vi "Autonomous Lift Gripper Pickup.vi"(8 "error in (no error)":errorcluster, 11 "Lift References":T19) -> (0 "error out":errorcluster, 3 "Lift References Out":T19)   [LabVIEW 2014]
uses:
  <vilib>/Rock Robotics/WPI/MotorControl/WPI_MotorControlDeviceRef.ctl
  <vilib>/Rock Robotics/WPI/MotorControl/WPI_MotorControlType.ctl
  <vilib>/Rock Robotics/SystemInterfaces/Typedef/FPGA_TypedefDigitalModule.ctl
  <vilib>/Rock Robotics/SystemInterfaces/DIO/FPGA_DIOPWMChannel.ctl
  <vilib>/Rock Robotics/WPI/PWM/WPI_PWMDeadband.ctl
  <vilib>/Rock Robotics/WPI/CAN/Jaguar/SubVIs/WPI_CANJaguar_ControlMode.ctl
  <vilib>/Rock Robotics/WPI/CAN/TalonSRX/WPI_CANTalonSRX_APIControlMode.ctl
  <vilib>/Rock Robotics/WPI/PWM/WPI_PWMTransform_ConPane.ctl
  <vilib>/Rock Robotics/WPI/Potentiometer/WPI_PotentiometerDevRef.ctl
  <vilib>/Rock Robotics/SystemInterfaces/Typedef/FPGA_TypedefAnalogModule.ctl
  <vilib>/Rock Robotics/SystemInterfaces/AI/FPGA_AIChannel.ctl
  <vilib>/Rock Robotics/WPI/Switch/WPI_SwitchDevRef.ctl
  <vilib>/Rock Robotics/SystemInterfaces/DIO/FPGA_DIOChannel.ctl
  <vilib>/Rock Robotics/SystemInterfaces/Counter/FPGA_CounterCtrSystemIndex.ctl
  <vilib>/Rock Robotics/WPI/Encoder/WPI_EncoderDevRef.ctl
  <vilib>/Rock Robotics/SystemInterfaces/Encoder/FPGA_EncoderIdx.ctl
  <vilib>/Rock Robotics/WPI/Encoder/WPI_EncoderType.ctl
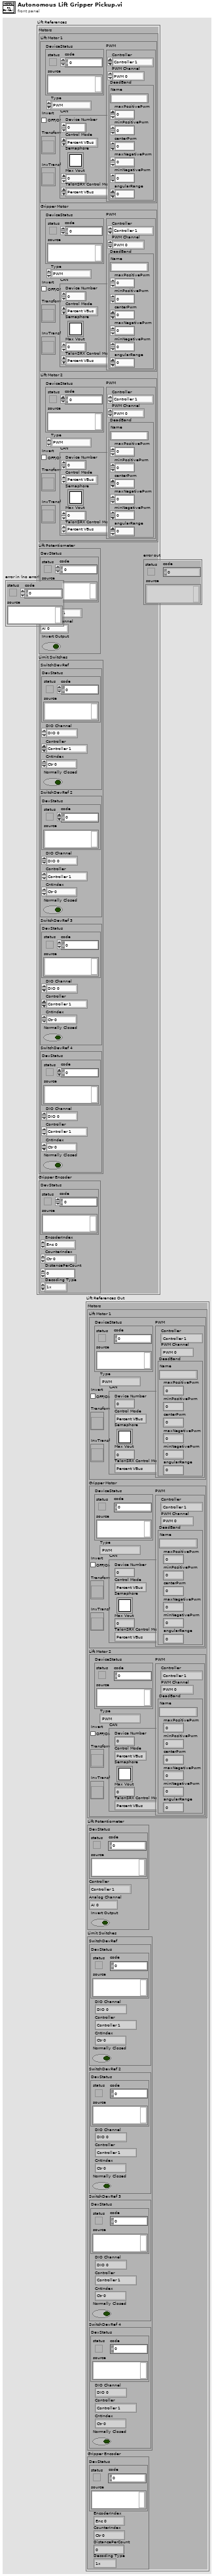
[diagram p1: front panel]
types:
  T1 = typedef "WPI_MotorControlDeviceRef.ctl" = cluster{"DeviceStatus":errorcluster, "Type":T2, "PWM":cluster{"Controller":T3, "PWM Channel":T4, "DeadBand":T5}, "CAN":cluster{"Device Number":u8, "Control Mode":T6, "Semaphore":T7, "Max Vout":dbl, "TalonSRX Control Mode":T8}, "Invert":bool, "TransformRef":T9, "InvTransformRef":T9}
  T2 = typedef "WPI_MotorControlType.ctl" = enum16{"PWM", "CAN", "CANTalonSRX"}
  T3 = typedef "FPGA_TypedefDigitalModule.ctl" = enum16{"Controller 1"}
  T4 = typedef "FPGA_DIOPWMChannel.ctl" = enum8{"PWM 0", "PWM 1", "PWM 2", "PWM 3", "PWM 4", "PWM 5", "PWM 6", "PWM 7", "PWM 8", "PWM 9", "PWM MXP 0", "PWM MXP 1", "PWM MXP 2", "PWM MXP 3", "PWM MXP 4", "PWM MXP 5", "PWM MXP 6", "PWM MXP 7", "PWM MXP 8", "PWM MXP 9", "Invalid"}
  T5 = typedef "WPI_PWMDeadband.ctl" = cluster{"Name":string, "maxPositivePwm":i32, "minPositivePwm":i32, "centerPwm":i32, "maxNegativePwm":i32, "minNegativePwm":i32, "angularRange":u16}
  T6 = typedef "WPI_CANJaguar_ControlMode.ctl" = enum8{"Percent VBus", "Current", "Speed", "Position", "Voltage"}
  T7 = typedef "Semaphore RefNum" = refnum<k1>
  T8 = typedef "WPI_CANTalonSRX_APIControlMode.ctl" = enum8{"Percent VBus", "Speed", "Position", "Slave", "Unchanged / Invalid"}
  T9 = typedef "WPI_PWMTransform_ConPane.ctl" = refnum<vi>
  T10 = typedef "WPI_PotentiometerDevRef.ctl" = cluster{"DevStatus":errorcluster, "Controller":T11, "Analog Channel":T12, "Invert Output":bool}
  T11 = typedef "FPGA_TypedefAnalogModule.ctl" = enum16{"Controller 1"}
  T12 = typedef "FPGA_AIChannel.ctl" = enum8{"AI 0", "AI 1", "AI 2", "AI 3", "AI MXP 0", "AI MXP 1", "AI MXP 2", "AI MXP 3", "Invalid"}
  T13 = typedef "WPI_SwitchDevRef.ctl" = cluster{"DevStatus":errorcluster, "DIO Channel":T14, "Controller":T3, "CntIndex":T15, "Normally Closed":bool}
  T14 = typedef "FPGA_DIOChannel.ctl" = enum8{"DIO 0", "DIO 1", "DIO 2", "DIO 3", "DIO 4", "DIO 5", "DIO 6", "DIO 7", "DIO 8", "DIO 9", "DIO MXP 0", "DIO MXP 1", "DIO MXP 2", "DIO MXP 3", "DIO MXP 4", "DIO MXP 5", "DIO MXP 6", "DIO MXP 7", "DIO MXP 8", "DIO MXP 9", "DIO MXP 10", "DIO MXP 11", "DIO MXP 12", "DIO MXP 13", "DIO MXP 14", "DIO MXP 15", "Invalid"}
  T15 = typedef "FPGA_CounterCtrSystemIndex.ctl" = enum8{"Ctr 0", "Ctr 1", "Ctr 2", "Ctr 3", "Ctr 4", "Ctr 5", "Ctr 6", "Ctr 7", "Invalid"}
  T16 = typedef "WPI_EncoderDevRef.ctl" = cluster{"DevStatus":errorcluster, "EncoderIndex":T17, "CounterIndex":T15, "DistancePerCount":dbl, "Decoding Type":T18}
  T17 = typedef "FPGA_EncoderIdx.ctl" = enum8{"Enc 0", "Enc 1", "Enc 2", "Enc 3", "Enc 4", "Enc 5", "Enc 6", "Enc 7", "Invalid"}
  T18 = typedef "WPI_EncoderType.ctl" = enum16{"1x", "2x", "4x"}
  T19 = cluster{"Motors":cluster{"Lift Motor 1":T1, "Gripper Motor":T1, "Lift Motor 2":T1}, "Lift Potentiometer":T10, "Limit Switches":cluster{"SwitchDevRef":T13, "SwitchDevRef 2":T13, "SwitchDevRef 3":T13, "SwitchDevRef 4":T13}, "Gripper Encoder":T16}
  T20 = cluster{"State Out":enum16{"Normal", "Down/Out", "Down/In", "Up", "Override"}, "To Shift":cluster{"Cluster in":cluster{"Scaled Value Out":dbl, "Distance":dbl}, "To Shift":cluster{"Error":dbl, "millisecond timer value":u32, "To Shift Register":dbl}, "To Shift":dbl}}
  T21 = cluster{"Lift Motor 1":T1, "Gripper Motor":T1, "Lift Motor 2":T1}
  T22 = cluster{"SwitchDevRef":T13, "SwitchDevRef 2":T13, "SwitchDevRef 3":T13, "SwitchDevRef 4":T13}
  T23 = enum16{"Normal", "Down/Out", "Down/In", "Up", "Override"}
  T24 = cluster{"Cluster in":cluster{"Scaled Value Out":dbl, "Distance":dbl}, "To Shift":cluster{"Error":dbl, "millisecond timer value":u32, "To Shift Register":dbl}, "To Shift":dbl}
  T25 = cluster{"Grabber Motor":T1, "Lift Motor 1":T1, "Lift Motor 2":T1}
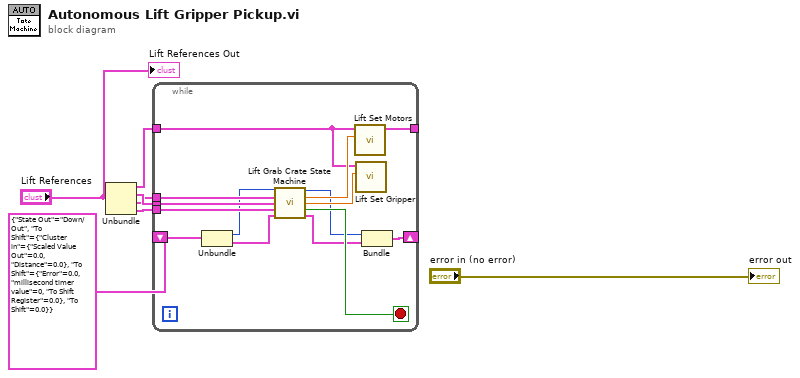
[diagram p0: block diagram]
diagram:
  n1 = Unbundle("Lift References") -> ("Motors"=w7:T21, "Lift Potentiometer"=w6:T10, "Limit Switches"=w5:T22, "Gripper Encoder"=w3:T16)
  n2 = while {
    shift-right: [w13] -> _
    shift-left: T20 {"State Out"=enum."Down/Out", "To Shift"={"Cluster in"={"Scaled Value Out"=0.0, "Distance"=0.0}, "To Shift"={"Error"=0.0, "millisecond timer value"=0, "To Shift Register"=0.0}, "To Shift"=0.0}} -> [w10]
    tunnel: w7 -> [w15]
    tunnel: w6 -> [w18]
    tunnel: w5 -> [w19]
    tunnel: w3 -> [w17]
    tunnel: [w14] -> _
    stop <- w21 stop-if-true
    n3 = Unbundle(w10) -> ("State Out"=w9:T23, "To Shift"=w8:T24)
    n4 = call "Lift Grab Crate State Machine.vi"("State In"=w9, "Limit Switches"=w19, "Lift Potentiometer"=w18, "Gripper Encoder"=w17, "From Shift"=w8) -> ("State Out"=w11:T23, "Lift Output"=w20:dbl, "Gripper Output"=w16:dbl, "Done?"=w21:bool, "To Shift"=w12:T24)  [unwired: 6 in]
    n5 = call "Lift Set Motors.vi"("Motor output"=w20, "Motors in"=w15) -> ("Motors out"=w14:T25)  [unwired: 8 in, 1 out]
    n6 = call "Lift Set Gripper.vi"("Motor output"=w16, "Motors in"=w15) -> ()  [unwired: 8 in, 2 out]
    n7 = Bundle("State Out"=w11, "To Shift"=w12) -> (w13:T20)  [unwired: 1 in]
  }
  "error out" <- "error in (no error)"
  "Lift References Out" <- "Lift References"
